vi "start.vi"(0 "TestSeries in":refnum<class "TestSeries.lvclass">, 5 "Serial Number":string, 7 "Operator":string, 9 "Comments":string, 11 "error in (no error)":errorcluster) -> (4 "TestSeries out":refnum<class "TestSeries.lvclass">, 15 "error out":errorcluster)   [LabVIEW 2016, in "TestSeries.lvclass"]
uses:
  TestSeries.lvclass
  Typedefs/TestLogTypes.ctl
  Typedefs/TestScenarioTypes.ctl
  TestSeries.lvclass/TestSeries.ctl
  abortTestSeries.vi
  TestLogFactory/ITestLogFactory/ITestLogFactory.lvclass
  TestLog/ITestLog/ITestLog.lvclass
  TestScenarioFactory/ITestScenarioFactory/ITestScenarioFactory.lvclass
  TestScenario/ITestScenario/ITestScenario.lvclass
  Typedefs/ILCBTTypedefs.lvlib
  Common_ILC/ILC/ILC.lvclass
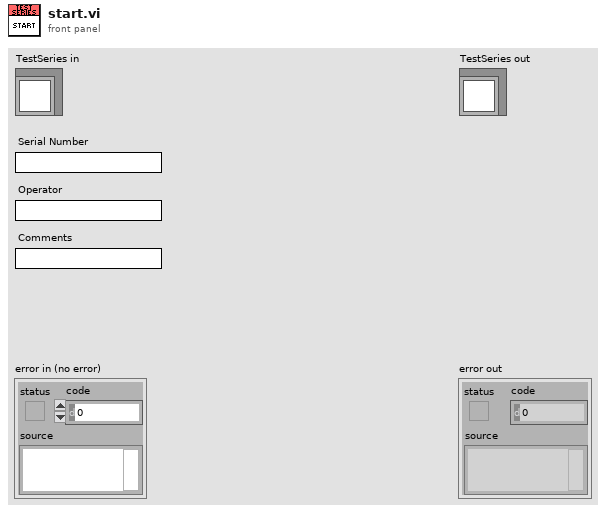
[diagram p1: front panel]
types:
  T1 = typedef "ILCBTTypedefs.lvlib/TestLogTypes.ctl" = enum16{"CSV Test Log"}
  T2 = typedef "ILCBTTypedefs.lvlib/TestScenarioTypes.ctl" = enum16{"+3.3VD", "+5.1V", "+24V", "RELVALV1", "RELVALV2", "Verify DAC_A = -1.00A", "Verify DAC_A = -0.75A", "Verify DAC_A = -0.50A", "Verify DAC_A = -0.25A", "Verify DAC_A = 0.00A", "Verify DAC_A = 0.25A", "Verify DAC_A = 0.50A", "Verify DAC_A = 0.75A", "Verify DAC_A = 1.00A", "Verify DAC_B = -1.00A", "Verify DAC_B = -0.75A", "Verify DAC_B = -0.50A", "Verify DAC_B = -0.25A", "Verify DAC_B = 0.00A", "Verify DAC_B = 0.25A", "Verify DAC_B = 0.50A", "Verify DAC_B = 0.75A", "Verify DAC_B = 1.00A", "Set DAC_A = -1.00A", "Set DAC_A = -0.75A", "Set DAC_A = -0.50A", "Set DAC_A = -0.25A", "Set DAC_A = 0.00A", "Set DAC_A = 0.25A", "Set DAC_A = 0.50A", "Set DAC_A = 0.75A", "Set DAC_A = 1.00A", "Set DAC_B = -1.00A", "Set DAC_B = -0.75A", "Set DAC_B = -0.50A", "Set DAC_B = -0.25A", "Set DAC_B = 0.00A", "Set DAC_B = 0.25A", "Set DAC_B = 0.50A", "Set DAC_B = 0.75A", "Set DAC_B = 1.00A", "Set MTR_PWR = On", "Set MTR_PWR = Off", "Set OUTPUT = On", "Set OUTPUT = Off", "Verify OUTPUT = On", "Verify OUTPUT = Off", "Verify POWER = Ok", "Verify POWER = Fail", "Verify AMP1 = Ok", "Verify AMP1 = Fail", "Verify AMP2 = Ok", "Verify AMP2 = Fail", "P1 0%", "P1 25%", "P1 50%", "P1 75%", "P1 100%", "P2 0%", "P2 25%", "P2 50%", "P2 75%", "P2 100%", "P3 0%", "P3 25%", "P3 50%", "P3 75%", "P3 100%", "P4 0%", "P4 25%", "P4 50%", "P4 75%", "P4 100%", "DCA 1 Linearity", "DCA 2 Linearity"}
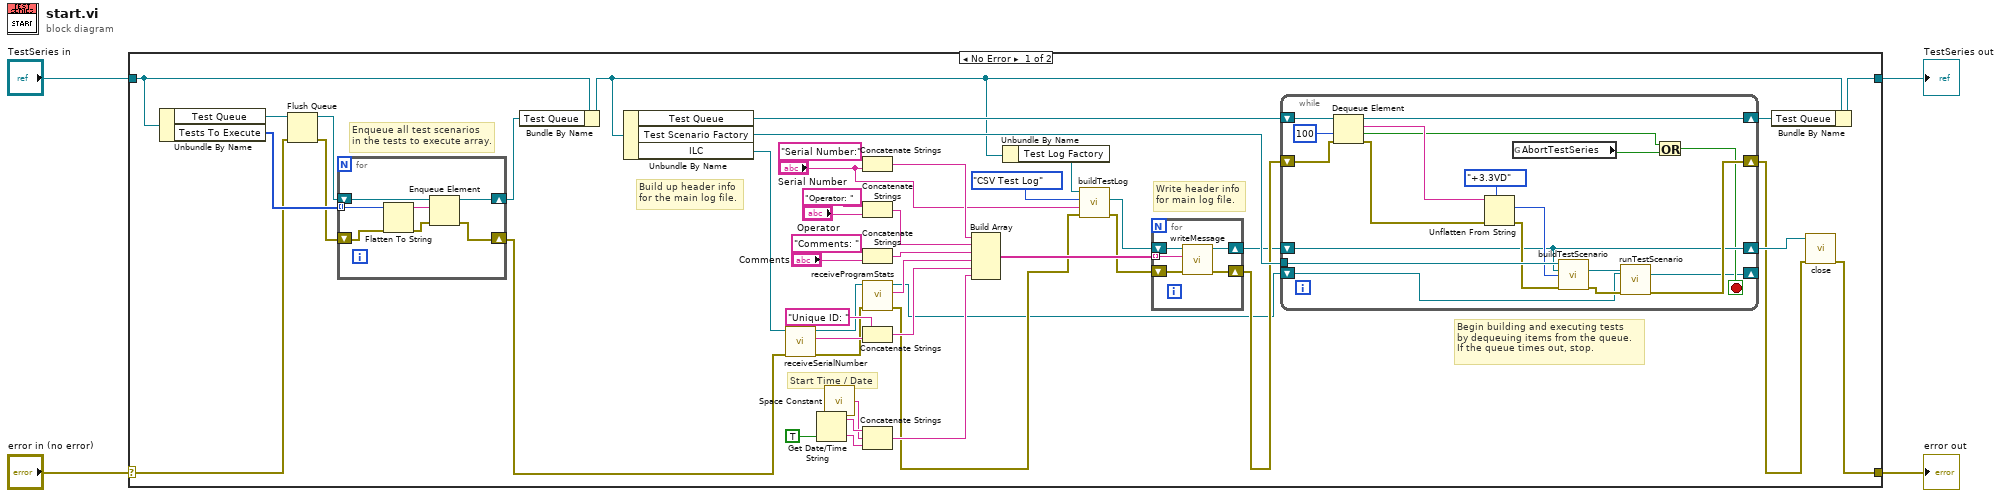
[diagram p0: block diagram]
diagram:
  n1 = case shown="No Error" "error in (no error)" {
    selector: "error in (no error)" -> [w45 w83]
    tunnel: [w7 w83] -> w3
    tunnel: [w41 w82] -> w1
    tunnel: "TestSeries in" -> [w49 w82]
    frame No Error {
      # "Begin building and executing tests\nby dequeuing items from the queue.\nIf the queue times out, stop."
      # "Write header info\nfor main log file."
      # "Build up header info\nfor the main log file."
      # "Enqueue all test scenarios\nin the tests to execute array."
      # "Start Time / Date"
      n2 = Unbundle By Name(w49) -> ("Test Queue"=w50:refnum<queue>, "Tests To Execute"=w48:T2[])
      n3 = Flush Queue(queue=w50, error in (no error)=w45) -> (queue out=w47:refnum<queue>, error out=w44:errorcluster)  [unwired: 1 out]
      n4 = for {
        tunnel: w48 -> [w57] mode=indexing
        shift-right: [w53] -> w46
        shift-left: w47 -> [w55]
        shift-right: [w51] -> w21
        shift-left: w44 -> [w52]
        n5 = Flatten To String(anything=w57, error in (no error)=w52) -> (data string=w56:string, error out=w54:errorcluster)  [unwired: 2 in, 1 out]
        n6 = Enqueue Element(queue=w55, element=w56, error in (no error)=w54) -> (queue out=w53:refnum<queue>, error out=w51:errorcluster)  [unwired: 1 in, 1 out]
      }
      n7 = Bundle By Name(cluster=w49, "Test Queue"=w46) -> (w18:refnum<class "TestSeries.lvclass">)
      n8 = Unbundle By Name(w18) -> ("Test Queue"=w43:refnum<queue>, "Test Scenario Factory"=w19:refnum<class "ITestScenarioFactory.lvclass">, "ILC"=w20:refnum<class "ILC.lvclass">)
      n9 = call "receiveSerialNumber.vi"("error in (no error)"=w21, "ILC in"=w20) -> ("error out"=w32:errorcluster, "Serial Number"=w40:string, "ILC out"=w33:refnum<class "ILC.lvclass">)  [unwired: 7 in]
      n10 = Get Date/Time String(want seconds? (F)=TRUE) -> (date string=w26:string, time string=w6:string)  [unwired: 2 in]
      n11 = call <vilib>:"Space Constant.vi"() -> ("String"=w25:string)
      n12 = Concatenate Strings("Serial Number:" ("string"), "Serial Number") -> (w31:string)
      n13 = Concatenate Strings("Operator: " ("string"), "Operator") -> (w30:string)
      n14 = Concatenate Strings("Comments: " ("string"), "Comments") -> (w29:string)
      n15 = call "receiveProgramStats.vi"("error in (no error)"=w32, "ILC in"=w33) -> ("error out"=w12:errorcluster, "Program Stats"=w28:string, "ILC out"=w5:refnum<class "ILC.lvclass">)  [unwired: 7 in]
      n16 = Concatenate Strings("Unique ID: " ("string"), w40) -> (w27:string)
      n17 = Concatenate Strings(w26, w25, w6) -> (w23:string)
      n18 = Build Array(w31, w30, w29, w28, w27, w23) -> (w22:string[])
      n19 = Unbundle By Name(w18) -> ("Test Log Factory"=w17:refnum<class "ITestLogFactory.lvclass">)
      n20 = call-dynamic "buildTestLog.vi"("error in (no error)"=w12, "Serial Number"="Serial Number", "TestLogTypes"=TestLogTypes."CSV Test Log", "ITestLogFactory in"=w17) -> ("error out"=w13:errorcluster, "ITestLog.lvclass"=w14:refnum<class "ITestLog.lvclass">)  [unwired: 5 in, 1 out]
      n21 = for {
        shift-right: [w58] -> w10
        shift-left: w14 -> [w61]
        tunnel: w22 -> [w60] mode=indexing
        shift-right: [w59] -> w11
        shift-left: w13 -> [w62]
        n22 = call-dynamic "writeMessage.vi"("error in (no error)"=w62, "Message"=w60, "ITestLog in"=w61) -> ("error out"=w59:errorcluster, "ITestLog out"=w58:refnum<class "ITestLog.lvclass">)  [unwired: 7 in]
      }
      n23 = while {
        shift-right: [w80] -> w42
        shift-left: w43 -> [w81]
        shift-right: [w69] -> w8
        shift-left: w11 -> [w78]
        tunnel: w19 -> [w77]
        shift-right: [w68] -> w9
        shift-left: w10 -> [w68]
        shift-right: [w63] -> _
        shift-left: w5 -> [w64]
        stop <- w65 stop-if-true
        n24 = Dequeue Element(queue=w81, timeout in ms (-1)=100, error in (no error)=w78) -> (queue out=w80:refnum<queue>, element=w75:string, timed out?=w66:bool, error out=w73:errorcluster)
        n25 = Unflatten From String(type=TestScenarioTypes."+3.3VD" ("Scenario"), binary string=w75, error in (no error)=w73) -> (value=w74:T2, error out=w72:errorcluster)  [unwired: 2 in, 1 out]
        n26 = global read "abortTestSeries.vi" "AbortTestSeries"() -> (w67:bool)
        n27 = call-dynamic "buildTestScenario.vi"("ITestScenarioFactory in"=w77, "Log"=w68, "Test Scenario"=w74, "error in (no error)"=w72) -> ("ITestScenario.lvclass"=w70:refnum<class "ITestScenario.lvclass">, "error out"=w71:errorcluster)  [unwired: 9 in, 1 out]
        n28 = call-dynamic "runTestScenario.vi"("ITestScenario in"=w70, "ILC"=w64, "error in (no error)"=w71) -> ("ILC 2"=w63:refnum<class "ILC.lvclass">, "error out"=w69:errorcluster)  [unwired: 8 in, 3 out]
        n29 = Or(x=w66, y=w67) -> (x .or. y?=w65:bool)
      }
      n30 = Bundle By Name(cluster=w18, "Test Queue"=w42) -> (w41:refnum<class "TestSeries.lvclass">)
      n31 = call-dynamic "close.vi"("error in (no error)"=w8, "ITestLog in"=w9) -> ("error out"=w7:errorcluster)  [unwired: 8 in, 1 out]
    }
    frame Error {
    }
  }
  "error out" <- w3
  "TestSeries out" <- w1
